vi "实验1-2.vi"() -> ()   [LabVIEW 2018]
panel:
  out "结果":dbl
  in  "数值c":dbl
  in  "数值b":dbl
  in  "数值a":dbl=4.0
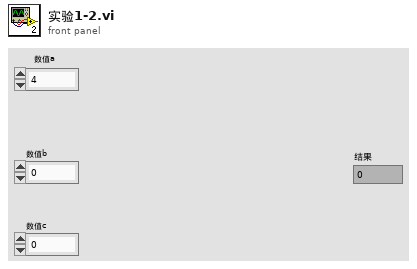
[diagram p1: front panel]
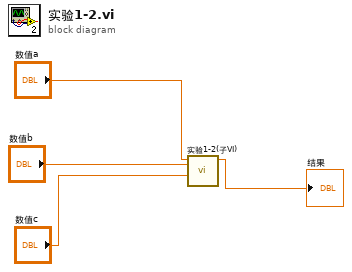
[diagram p0: block diagram]
diagram:
  n1 = call "实验1-2(子VI).vi"("数值c"="数值c", "数值b"="数值b", "数值a"="数值a") -> ("结果"=→"结果":dbl)  [unwired: 8 in]
